vi "HFRR ADV v07.vi"() -> ()   [LabVIEW 2025] (continued)
                n1812 = local read "TEMPERATURE :"() -> (w2456:dbl)
                n1813 = local read "FRIC. FORCE :"() -> (w2457:dbl)
                n1814 = local read "HUMIDITY:"() -> (w2454:dbl)
                n1815 = Path To String(path="File Path") -> (string=w2524:string)
                n1816 = Number To Fractional String(number=w2463, width (-)=i16 10 ("precision (6)"), precision (6)=i16 5) -> (F-format string=w2482:string)  [unwired: 1 in]
                n1817 = Number To Fractional String(number=w2466, width (-)=i16 10 ("precision (6)"), precision (6)=i16 5) -> (F-format string=w2487:string)  [unwired: 1 in]
                n1818 = Number To Fractional String(number=w2469, width (-)=i16 10 ("precision (6)"), precision (6)=i16 5) -> (F-format string=w2490:string)  [unwired: 1 in]
                n1819 = Number To Fractional String(number=w2472, width (-)=i16 10 ("precision (6)"), precision (6)=i16 5) -> (F-format string=w2495:string)  [unwired: 1 in]
                n1820 = Number To Fractional String(number=w2475, width (-)=i16 10 ("precision (6)"), precision (6)=i16 5) -> (F-format string=w2498:string)  [unwired: 1 in]
                n1821 = Number To Fractional String(number=w2508, width (-)=i16 10 ("precision (6)"), precision (6)=i16 5) -> (F-format string=w2504:string)  [unwired: 1 in]
                n1822 = Number To Fractional String(number=w2452, width (-)=i16 10 ("precision (6)"), precision (6)=i16 5) -> (F-format string=w2515:string)  [unwired: 1 in]
                n1823 = local read "Com Port 2"() -> (w2458:refnum<visa-resource-name>)
                n1824 = local read "Com Port 1"() -> (w2459:refnum<visa-resource-name>)
                n1825 = Concatenate Strings(w2524, "\\" ("string")) -> (w2523:string)
                n1826 = Number To Fractional String(number=w2453, width (-)=i16 10 ("precision (6)"), precision (6)=i16 5) -> (F-format string=w2516:string)  [unwired: 1 in]
                n1827 = Number To Fractional String(number=w2455, width (-)=i16 10 ("precision (6)"), precision (6)=i16 5) -> (F-format string=w2543:string)  [unwired: 1 in]
                n1828 = Number To Fractional String(number=w2454, width (-)=i16 10 ("precision (6)"), precision (6)=i16 5) -> (F-format string=w2549:string)  [unwired: 1 in]
                n1829 = Number To Fractional String(number=w2456, width (-)=i16 10 ("precision (6)"), precision (6)=i16 5) -> (F-format string=w2555:string)  [unwired: 1 in]
                n1830 = Number To Fractional String(number=w2457, width (-)=i16 10 ("precision (6)"), precision (6)=i16 5) -> (F-format string=w2556:string)  [unwired: 1 in]
                n1831 = Concatenate Strings("[CHH]" ("string"), w2482, "-Humidity Dry" ("string"), "\r") -> (w2476:string)
                n1832 = Concatenate Strings("[CHG]" ("string"), w2487, "-Humidity Wet" ("string"), "\r") -> (w2477:string)
                n1833 = Concatenate Strings("[CHD]" ("string"), w2498, "-Power +" ("string"), "\r") -> (w2480:string)
                n1834 = Concatenate Strings("[CHC]" ("string"), w2504, "-Language Selection" ("string"), "\r") -> (w2501:string)
                n1835 = Concatenate Strings("[CHA]" ("string"), w2515, "- Stroke Gain" ("string"), "\r") -> (w2509:string)
                n1836 = Concatenate Strings("[CHF]" ("string"), w2490, "-Heater" ("string"), "\r") -> (w2478:string)
                n1837 = Concatenate Strings("[CHE]" ("string"), w2495, "-Power_" ("string"), "\r") -> (w2479:string)
                n1838 = Concatenate Strings("[CH8]" ("string"), w2516, "- Displacement Gain" ("string"), "\r") -> (w2519:string)
                n1839 = Concatenate Strings("[CH7]" ("string"), w2523, "- file path" ("string"), "\r") -> (w2526:string)
                n1840 = Concatenate Strings("[CH6]" ("string"), w2458, "- Visa Due" ("string"), "\r") -> (w2527:string)
                n1841 = Concatenate Strings("[CH5]" ("string"), w2459, "- Visa Uno" ("string"), "\r") -> (w2532:string)
                n1842 = Concatenate Strings("[CH4]" ("string"), w2543, " - AIR TEMP" ("string"), "\r") -> (w2539:string)
                n1843 = Concatenate Strings("[CH3]" ("string"), w2549, " - Humidity" ("string"), "\r") -> (w2546:string)
                n1844 = Concatenate Strings("[CH2]" ("string"), w2555, " - TEMPERATURE" ("string"), "\r") -> (w2553:string)
                n1845 = Concatenate Strings("[CH1]" ("string"), w2556, " - FF" ("string"), "\r") -> (w2554:string)
                n1846 = Concatenate Strings(w2554, w2553, w2546, w2539, w2532, w2527, w2526, w2519, w2509, w2501, w2480, w2479, w2478, w2477, w2476) -> (w2460:string)
                "gain" <- w2460
              }
              frame #1 {
                n1847 = local read "Camera Port :"() -> (w2568:string)
                n1848 = local read "C3 :"() -> (w2576:refnum<visa-resource-name>)
                n1849 = local read "TEMP INTERCEPT:"() -> (w2577:dbl)
                n1850 = local read "AIR TEMP INTERCEPT:"() -> (w2578:dbl)
                n1851 = Concatenate Strings("[CH8]" ("string"), w2568, "- Visa Camera" ("string"), "\r") -> (w2567:string)
                n1852 = Concatenate Strings("[CH7]" ("string"), w2576, "- Visa Humidity" ("string"), "\r") -> (w2572:string)
                n1853 = Number To Fractional String(number=w2577, width (-)=i16 10 ("precision (6)"), precision (6)=i16 5) -> (F-format string=w2595:string)  [unwired: 1 in]
                n1854 = local read "Com Port 3"() -> (w2579:refnum<visa-resource-name>)
                n1855 = Number To Fractional String(number=w2578, width (-)=i16 10 ("precision (6)"), precision (6)=i16 5) -> (F-format string=w2602:string)  [unwired: 1 in]
                n1856 = Concatenate Strings("[SNO]" ("string"), "S.NO", "-" ("string"), "\r") -> (w2587:string)
                n1857 = Concatenate Strings("[CHK]" ("string"), w2595, "-TEMP INTERCEPT" ("string"), "\r") -> (w2591:string)
                n1858 = Concatenate Strings("[CHJ]" ("string"), w2602, "-AIR TEMP INTERCEPT" ("string"), "\r") -> (w2592:string)
                n1859 = Concatenate Strings("[CHL]" ("string"), w2579, "- Visa humid" ("string"), "\r") -> (w2582:string)
                n1860 = String To Path(string="C:\\LAB-IQ\\calibrate WO 2465.dcf") -> (path=w2580:path)
                n1861 = Concatenate Strings(w2607, w2592, w2591, w2587, w2582, w2572, w2567) -> (w2606:string)
                n1862 = call <vilib>:"Write Characters To File.vi"("append to file? (new file:F)"=FALSE, "character string"=w2606, "file path (dialog if empty)"=w2580) -> ()  [unwired: 2 in, 1 out]
              }
              frame #2 {
                n1863 = local write "Lan flag"(0.0 ("Lan flag")) -> ()
                n1864 = local write "conststatus"(0.0 ("rpm value : 2")) -> ()
                n1865 = local write "SAVE"(FALSE ("OK Button 14")) -> ()
                n1866 = local write "SAVE 2"(FALSE ("SAVE 2")) -> ()
              }
            }
          }
        }
        n1867 = property on="Tab Control 7" class="TabCtl (strict)"("Disabled"=w2247) -> ()  [unwired: 2 in, 2 out]
        n1868 = property on="TEMP INTERCEPT:" class="DigNum (strict)"("Disabled"=w2247) -> ()  [unwired: 2 in, 2 out]
        n1869 = property on="AIR TEMP INTERCEPT:" class="DigNum (strict)"("Disabled"=w2247) -> ()  [unwired: 2 in, 2 out]
        n1870 = property on="DISPLACEMENT :" class="DigNum (strict)"("Disabled"=w2247) -> ()  [unwired: 2 in, 2 out]
        n1871 = property on="STROKE GAIN :" class="DigNum (strict)"("Disabled"=w2247) -> ()  [unwired: 2 in, 2 out]
        n1872 = property on="CH-HUMIDITY DRY" class="DigNum (strict)"("Disabled"=w2247) -> ()  [unwired: 2 in, 2 out]
        n1873 = property on="CH-HUMIDITY WET" class="DigNum (strict)"("Disabled"=w2247) -> ()  [unwired: 2 in, 2 out]
        n1874 = property on="CH-HEATER" class="DigNum (strict)"("Disabled"=w2247) -> ()  [unwired: 2 in, 2 out]
        n1875 = property on="CH-POWER -" class="DigNum (strict)"("Disabled"=w2247) -> ()  [unwired: 2 in, 2 out]
        n1876 = property on="CH-POWER +" class="DigNum (strict)"("Disabled"=w2247) -> ()  [unwired: 2 in, 2 out]
        n1877 = property on="Language Selection" class="Enum (strict)"("Visible"=w2246) -> ()  [unwired: 2 in, 2 out]
        n1878 = property on="AIR TEMPERATURE :" class="DigNum (strict)"("Disabled"=w2247) -> ()  [unwired: 2 in, 2 out]
        n1879 = property on="HUMIDITY:" class="DigNum (strict)"("Disabled"=w2247) -> ()  [unwired: 2 in, 2 out]
        n1880 = property on="FRIC. FORCE :" class="DigNum (strict)"("Disabled"=w2247) -> ()  [unwired: 2 in, 2 out]
        n1881 = property on="TEMPERATURE :" class="DigNum (strict)"("Disabled"=w2247) -> ()  [unwired: 2 in, 2 out]
        n1882 = property on="SPEED OUT:" class="DigNum (strict)"("Disabled"=w2247) -> ()  [unwired: 2 in, 2 out]
      }
    }
    n1883 = case shown="False" w1641 {
      frame False {
        n1884 = local read "stopT"() -> (w2619:bool)
        n1885 = case shown="True" w2619 {
          frame False {
          }
          frame True {
            n1886 = local write "stopT"(FALSE) -> ()
          }
        }
      }
      frame True {
        "stopT" <- TRUE
      }
    }
    n1887 = case shown="True" w1629 {
      frame False {
        n1888 = property on="Password 2" class="Str"("Visible"=FALSE) -> ()  [unwired: 2 in, 2 out]
        n1889 = local write "Password 2"("" ("Password")) -> ()
      }
      frame True {
        n1890 = property on="Password 2" class="Str"("Visible"=TRUE) -> ()  [unwired: 2 in, 2 out]
        n1891 = Equal?(x="Password 2", y="HFRR1234") -> (x = y?=w1761:bool)
        n1892 = case shown="True" w1761 {
          tunnel: "Password 2" -> [w1764 _]
          frame False {
            n1893 = String Length(string=w1764) -> (length=w1765:i32)
            n1894 = Greater Than 0?(x=w1765) -> (x > 0?=w1763:bool)
            n1895 = case shown="False" w1763 {
              frame False {
                n1896 = property on="Password 2" class="Str"("Caption.Text"="Password (Advance Setting)") -> ()  [unwired: 2 in, 2 out]
              }
              frame True {
                n1897 = property on="Password 2" class="Str"("Caption.Text"="Incorrect Password!") -> ()  [unwired: 2 in, 2 out]
              }
            }
          }
          frame True {
            (unwired) T26."Advance" ("Main Dashboard Buttons")
            n1898 = local write "EDIT 2"(FALSE ("EDIT 2")) -> ()
            n1899 = local write "Password 2"("" ("Password")) -> ()
            n1900 = local write "Main Tab"(T2."Advance" ("Main Tab")) -> ()
            n1901 = local write "Main Dashboard Buttons"(T1."Advance" ("Main Dashboard Buttons")) -> ()
          }
        }
      }
    }
    n1902 = disable-structure shown="Disabled" {
      disable-tunnel: [w1656 _] -> w1622
      disable-tunnel: [w1655 _] -> w1620
      frame Disabled {
        n1903 = local read "Temperature before test"() -> (w1649:dbl)
        n1904 = local read "Temperature after test"() -> (w1662:dbl)
        n1905 = Add(x=231.864, y=w1662) -> (x+y=w1659:dbl)
        n1906 = Add(x=231.864, y=w1649) -> (x+y=w1646:dbl)
        n1907 = case shown="True" "Save Results" {
          frame False {
          }
          frame True {
            w1678 = "\r"
            n1908 = local write "Save Results"(FALSE ("OK Button 5")) -> ()
            n1909 = local read "Temperature before test"() -> (w1716:dbl)
            n1910 = local read "Temperature after test"() -> (w1718:dbl)
            n1911 = local read "Humidity before test"() -> (w1715:dbl)
            n1912 = local read "Humidity after test"() -> (w1717:dbl)
            n1913 = local read "WS1.4"() -> (w1722:dbl)
            n1914 = local read "AVP"() -> (w1720:dbl)
            n1915 = Number To Fractional String(number=w1722, width (-)=i16 6, precision (6)=i16 1) -> (F-format string=w1682:string)  [unwired: 1 in]
            n1916 = local read "MWSD"() -> (w1719:dbl)
            n1917 = local read "String"() -> (w1711:string)
            n1918 = local read "FILE"() -> (w1714:string)
            n1919 = local read "HCF"() -> (w1721:dbl)
            n1920 = Number To Fractional String(number=w1718, width (-)=i16 6, precision (6)=i16 1) -> (F-format string=w1696:string)  [unwired: 1 in]
            n1921 = Number To Fractional String(number=w1717, width (-)=i16 6, precision (6)=i16 1) -> (F-format string=w1700:string)  [unwired: 1 in]
            n1922 = Number To Fractional String(number=w1720, width (-)=i16 6, precision (6)=i16 3) -> (F-format string=w1689:string)  [unwired: 1 in]
            n1923 = Number To Fractional String(number=w1716, width (-)=i16 6, precision (6)=i16 1) -> (F-format string=w1704:string)  [unwired: 1 in]
            n1924 = Number To Fractional String(number=w1715, width (-)=i16 6, precision (6)=i16 1) -> (F-format string=w1707:string)  [unwired: 1 in]
            n1925 = Concatenate Strings(w1711, w1714) -> (w1733:string)
            n1926 = Number To Fractional String(number=w1721, width (-)=i16 6, precision (6)=i16 2) -> (F-format string=w1687:string)  [unwired: 1 in]
            n1927 = Number To Fractional String(number=w1719, width (-)=i16 6, precision (6)=i16 1) -> (F-format string=w1693:string)  [unwired: 1 in]
            n1928 = Concatenate Strings("(" ("string"), w1682, ")Microns" ("string")) -> (w1681:string)
            n1929 = local read "REMARKS"() -> (w1713:string)
            "REMARKS 2" <- w1713
            n1930 = Concatenate Strings(w1687, ")" ("string")) -> (w1685:string)
            n1931 = Concatenate Strings("(" ("string"), w1707, " ) % RH," ("string")) -> (w1708:string)
            n1932 = Concatenate Strings("(" ("string"), w1689, ")  kPa," ("string")) -> (w1679:string)
            n1933 = Concatenate Strings("(" ("string"), w1693, ")  Microns," ("string")) -> (w1692:string)
            n1934 = Concatenate Strings("(" ("string"), w1696, ")  Deg C ," ("string")) -> (w1695:string)
            n1935 = Concatenate Strings("(" ("string"), w1700, " ) % RH," ("string")) -> (w1699:string)
            n1936 = Concatenate Strings("(" ("string"), w1704, ")  Deg C ," ("string")) -> (w1703:string)
            n1937 = Concatenate Strings(w1733, ".dwm" ("Substring")) -> (w1731:string)
            n1938 = String To Path(string=w1731) -> (path=w1730:path)
            n1939 = Concatenate Strings(w1713, w1678, " Humidity before test= " ("Substring"), w1708, w1678, " Temperature before test = " ("Substring"), w1703, w1678, " Humidity after test= " ("Substring"), w1699, w1678, "Temperature after test = " ("Substring"), w1695, w1678, "MSD = " ("Substring"), w1692, w1678, "  AVP = " ("Substring"), w1679, w1678, "  HCF                     =( " ("Substring"), w1685, w1678, " WS1.4                  = " ("Substring"), w1681, w1678) -> (w1677:string)
            "data" <- w1677
            n1940 = call <vilib>:"Write Characters To File.vi"("append to file? (new file:F)"=FALSE, "character string"=w1677, "file path (dialog if empty)"=w1730) -> ()  [unwired: 2 in, 1 out]
            n1941 = Match Pattern(string=w1677, regular expression="!") -> (after substring=→"export":string)  [unwired: 1 in, 3 out]
          }
        }
        n1942 = Divide(x=1705.984, y=w1659) -> (x/y=w1660:dbl)
        n1943 = Divide(x=1705.984, y=w1646) -> (x/y=w1647:dbl)
        n1944 = local read "Humidity before test"() -> (w1651:dbl)
        n1945 = local read "Humidity after test"() -> (w1664:dbl)
        n1946 = Subtract(x=8.017352 ("y"), y=w1660) -> (x-y=w1667:dbl)
        n1947 = Subtract(x=8.017352 ("y"), y=w1647) -> (x-y=w1673:dbl)
        n1948 = expression code="10**y"(w1667) -> (w1666:dbl)
        n1949 = expression code="10**y"(w1673) -> (w1653:dbl)
        n1950 = Multiply(x=w1664, y=w1666) -> (x*y=w1665:dbl)
        n1951 = Multiply(x=w1651, y=w1653) -> (x*y=w1652:dbl)
        n1952 = Divide(x=w1665, y=750.0) -> (x/y=w1669:dbl)
        n1953 = Divide(x=w1652, y=750.0) -> (x/y=w1668:dbl)
        n1954 = Add(x=w1668, y=w1669) -> (x+y=w1670:dbl)
        n1955 = Divide(x=w1670, y=2.0) -> (x/y=w1672:dbl)
        n1956 = local write "AVP"(w1672) -> ()
        n1957 = Subtract(x=1.4, y=w1672) -> (x-y=w1655:dbl)
        n1958 = local read "HCF"() -> (w1656:dbl)
      }
      frame Enabled {
      }
    }
    n1959 = case shown="\"Acquire\", Default" w1637 {
      frame "Acquire", Default {
        w2650 = 0.2 ("y")
        w2655 = 1.0 ("y")
        w2656 = 0.8 ("y")
        # "Elapsed time\ncof\nstroke\nAir temp\nTemp\nHumidity"
        n1960 = local read "RUN"() -> (w2659:bool)
        n1961 = local read "run replace"() -> (w2663:bool)
        n1962 = local read "run replace"() -> (w2662:bool)
        n1963 = stacked-sequence {
          frame #0 {
            n1964 = case shown="True" "RST FF" {
              frame False {
              }
              frame True {
                w2831 = 0.0 ("X Scale.Range:Maximum")
                n1965 = property on="Frictional Force ( N )" class="WFChart (strict)"("XScale.Maximum"=600.0 ("X Scale.Range:Maximum"), "XScale.Minimum"=w2831, "YScale.Maximum"=10.0 ("Y Scale.Range:Maximum"), "YScale.Minimum"=w2831) -> ()  [unwired: 2 in, 2 out]
              }
            }
          }
          frame #1 {
            n1966 = case shown="True" "RST TEMP" {
              frame False {
              }
              frame True {
                n1967 = property on="Temperature ( Deg C )" class="WFChart (strict)"("XScale.Minimum"=0.0 ("X Scale.Range:Minimum"), "XScale.Maximum"=600.0 ("X Scale.Range:Maximum"), "YScale.Minimum"=0.0 ("Y Scale.Range:Minimum"), "YScale.Maximum"=100.0 ("Y Scale.Range:Maximum")) -> ()  [unwired: 2 in, 2 out]
              }
            }
          }
          frame #2 {
            n1968 = case shown="True" "RSTCOF" {
              frame False {
              }
              frame True {
                n1969 = property on="Coefficient of Friction" class="WFChart (strict)"("XScale.Minimum"=0.0 ("X Scale.Range:Minimum"), "XScale.Maximum"=600.0 ("X Scale.Range:Maximum"), "YScale.Maximum"=1.0 ("X Scale.Range:Minimum"), "YScale.Minimum"=0.0 ("X Scale.Range:Minimum")) -> ()  [unwired: 2 in, 2 out]
              }
            }
          }
          frame #3 {
            n1970 = case shown="True" "RSTCOF 2" {
              frame False {
              }
              frame True {
                (unwired) 100.0 ("Y Scale.Range:Maximum")
                (unwired) 0.0 ("Y Scale.Range:Minimum")
                (unwired) 600.0 ("X Scale.Range:Maximum")
                (unwired) 0.0 ("X Scale.Range:Minimum")
              }
            }
          }
          frame #4 {
            n1971 = case shown="True" "RSTCOF 3" {
              frame False {
              }
              frame True {
                n1972 = property on="Electrical Contact Resistance ( % )" class="WFChart (strict)"("XScale.Minimum"=0.0 ("X Scale.Range:Minimum"), "XScale.Maximum"=600.0 ("X Scale.Range:Maximum"), "YScale.Minimum"=0.0 ("Y Scale.Range:Minimum"), "YScale.Maximum"=100.0 ("Y Scale.Range:Maximum")) -> ()  [unwired: 2 in, 2 out]
              }
            }
          }
        }
        n1973 = case shown="True" w2659 {
          frame False {
            n1974 = local write "run replace"(FALSE ("run replace")) -> ()
          }
          frame True {
            "run replace" <- TRUE ("run replace")
          }
        }
        n1975 = disable-structure shown="Disabled" {
          frame Disabled {
            n1976 = local read "RUN"() -> (w2670:bool)
            n1977 = local read "Flag"() -> (w2673:dbl)
            n1978 = Not(x=w2670) -> (.not. x?=w2669:bool)
            n1979 = Equal?(x=w2673, y=10.0) -> (x = y?=w2671:bool)
            n1980 = And(x=w2671, y=w2669) -> (x .and. y?=w2668:bool)
            n1981 = case shown="True" w2668 {
              frame False {
              }
              frame True {
                w2674 = FALSE ("Heater Button")
                n1982 = local write "Humidity"(w2674) -> ()
                n1983 = local write "Heater Button"(w2674) -> ()
              }
            }
          }
          frame Enabled {
          }
        }
        n1984 = local read "RUN"() -> (w2667:bool)
        n1985 = local read "Set Temp"() -> (w2629:dbl)
        n1986 = local read "SetTemp"() -> (w2631:dbl)
        n1987 = case shown="False" w2667 {
          tunnel: [FALSE ("TEST RUNNING") TRUE ("TEST RUNNING")] -> w2666
          frame False {
            w2850 = 0.0 ("Flag")
            n1988 = local write "Elapsed time"(0.0 ("elapsedtime")) -> ()
            n1989 = local write "Time Remaining"(w2850) -> ()
            n1990 = local write "Flag"(w2850) -> ()
            n1991 = local write "Remaining Time"(w2850) -> ()
          }
          frame True {
            n1992 = local write "Flag"(10.0 ("Flag")) -> ()
          }
        }
        n1993 = case shown="False" w2663 {
          frame False {
            n1994 = local read "zflag"() -> (→"zflag 2":dbl)
            n1995 = local write "FLAG 4"(0.0 ("FLAG")) -> ()
            n1996 = local write "yflag"(2.0 ("tflag")) -> ()
          }
          frame True {
            n1997 = local write "zflag"(3.0 ("zflag")) -> ()
            n1998 = local write "yflag"(1.0 ("tflag")) -> ()
          }
        }
        n1999 = local read "acq 2"() -> (w2661:bool)
        n2000 = local read "AIR TEMP"() -> (w2624:dbl)
        n2001 = local read "Amb temp"() -> (w2628:dbl)
        n2002 = case shown="True" "Save & Continue" {
          frame False {
          }
          frame True {
            "acq 2" <- TRUE ("acq 2")
          }
        }
        n2003 = local read "Set Rh"() -> (w2630:dbl)
        n2004 = Subtract(x=w2629, y=w2650) -> (x-y=w2652:dbl)
        n2005 = Add(x=w2629, y=w2650) -> (x+y=w2651:dbl)
        n2006 = Subtract(x=w2631, y=w2656) -> (x-y=w2658:dbl)
        n2007 = Add(x=w2631, y=w2656) -> (x+y=w2657:dbl)
        n2008 = And(x=w2661, y=w2662) -> (x .and. y?=w2660:bool)
        n2009 = disable-structure shown="Disabled" {
          frame Disabled {
            n2010 = case shown="True" {
              selector: _ -> [_ _]
              frame False {
              }
              frame True {
                n2011 = local read "zflag 2"() -> (w2732:dbl)
                n2012 = local read "yflag"() -> (w2734:dbl)
                n2013 = Equal?(x=w2732, y=3.0 ("tflag")) -> (x = y?=w2735:bool)
                n2014 = Equal?(x=w2734, y=2.0 ("tflag")) -> (x = y?=w2736:bool)
                n2015 = And(x=w2736, y=w2735) -> (x .and. y?=w2730:bool)
                n2016 = case shown="True" w2730 {
                  frame False {
                  }
                  frame True {
                    w2761 = 0.0 ("zflag")
                    n2017 = local write "zflag 2"(w2761) -> ()
                    n2018 = local write "zflag"(w2761) -> ()
                    n2019 = Delete(path (use dialog)=path "C:/LAB-IQ-NXT/WO 2449 TT.sig" ("file path (dialog if empty)")) -> (deleted path=w2760:path)  [unwired: 4 in, 2 out]
                    n2020 = Delete(path (use dialog)=path "C:/LAB-IQ-NXT/WO 2449 TRH.sig" ("file path (dialog if empty)")) -> (deleted path=w2755:path)  [unwired: 4 in, 2 out]
                    n2021 = local read "SENSOR TIME"() -> (w2745:dbl)
                    n2022 = local read "SEN.RUN HRS"() -> (w2747:dbl)
                    n2023 = call <vilib>:"compatOverwrite.vi"("overwrite (F)"=TRUE) -> ("overwrite?"=w2737:T27)
                    n2024 = call <vilib>:"compatOverwrite.vi"("overwrite (F)"=TRUE) -> ("overwrite?"=w2741:T27)
                    n2025 = local read "Total No. of Tests"() -> (w2748:dbl)
                    n2026 = Add(x=w2745, y=w2747) -> (x+y=w2746:dbl)
                    "SEN.RUN HRS" <- w2746
                    n2027 = Open/Create/Replace File(file path (use dialog)=w2760, operation (0:open)=w2737) -> (refnum out=w2738:refnum<file>, error out=w2739:errorcluster)  [unwired: 4 in, 1 out]
                    n2028 = Open/Create/Replace File(file path (use dialog)=w2755, operation (0:open)=w2741) -> (refnum out=w2742:refnum<file>, error out=w2743:errorcluster)  [unwired: 4 in, 1 out]
                    n2029 = Deny Access(4:w2739, 6:T24."deny none" ("deny mode (2)"), 7:w2738) -> (3:w2759:refnum<file>)  [unwired: 1 out]
                    n2030 = Deny Access(4:w2743, 6:T24."deny none" ("deny mode (2)"), 7:w2742) -> (3:w2751:refnum<file>)  [unwired: 1 out]
                    n2031 = Number To Decimal String(number=w2748) -> (decimal integer string=w2756:string)  [unwired: 1 in]
                    n2032 = Number To Decimal String(number=w2746) -> (decimal integer string=w2752:string)  [unwired: 1 in]
                    n2033 = Write to Binary File(file (use dialog)=w2759, data=w2756, 5:FALSE ("prepend array or string size? (T)")) -> ()  [unwired: 3 in, 3 out]
                    n2034 = Write to Binary File(file (use dialog)=w2751, data=w2752, 5:FALSE ("prepend array or string size? (T)")) -> ()  [unwired: 3 in, 3 out]
                  }
                }
              }
            }
          }
          frame Enabled {
          }
        }
        n2035 = Greater Or Equal?(x=w2624, y=15.0) -> (x >= y?=w2625:bool)
        "powstat" <- w2625
        n2036 = local read "Humidity ( %RH )"() -> (w2627:dbl)
        n2037 = Subtract(x=w2630, y=w2655) -> (x-y=w2653:dbl)
        n2038 = Add(x=w2630, y=w2655) -> (x+y=w2654:dbl)
        n2039 = In Range and Coerce(upper limit=w2657, x=w2628, lower limit=w2658) -> (In Range?=w2647:bool)  [unwired: 1 out]
        n2040 = local read "TEMP"() -> (w2626:dbl)
        n2041 = case shown="True" "Save & Continue" {
          frame False {
          }
          frame True {
            n2042 = local read "Operator ID"() -> (w3130:string)
            n2043 = local read "FILE"() -> (w3136:string)
            n2044 = String Length(string=w3130) -> (length=w3131:i32)
            n2045 = String Length(string=w3136) -> (length=w3134:i32)
            n2046 = Greater?(x=w3131, y=0) -> (0:w3129:bool)
            n2047 = Greater?(x=w3134, y=0) -> (0:w3133:bool)
            n2048 = And(x=w3133, y=w3129) -> (x .and. y?=w3128:bool)
            n2049 = case shown="True" w3128 {
              frame False {
                n2050 = stacked-sequence {
                  frame #0 {
                    n2051 = One Button Dialog(message="Please Enter a File Name and Operator ID to save data !", button name ("OK")="Ok") -> ()  [unwired: 1 out]
                  }
                  frame #1 {
                    n2052 = local write "Save & Continue"(FALSE ("OK Button")) -> ()
                  }
                }
                n2053 = local write "Save & Continue"(FALSE ("OK Button")) -> ()
              }
              frame True {
                n2054 = stacked-sequence {
                  frame #0 {
                    n2055 = local read "FILE"() -> (w3142:string)
                    n2056 = call "file check.vi"("file name in"=w3142) -> ("file name out"=w3141:string)  [unwired: 9 in, 1 out]
                    n2057 = call <vilib>:"Application Directory.vi"() -> ("Application Directory"=w3152:path)
                    n2058 = Build Path(base path=w3152, name or relative path="data") -> (appended path=w3151:path)
                    n2059 = call <vilib>:"Trim Whitespace.vi"("string"=w3141) -> ("trimmed string"=w3149:string)  [unwired: 1 in]
                    n2060 = call <vilib>:"Trim Whitespace.vi"("string"=w3141) -> ("trimmed string"=w3150:string)  [unwired: 1 in]
                    n2061 = List Folder(path=w3151) -> (folder names=w3147:string[])  [unwired: 3 in, 3 out]
                    n2062 = Match Pattern(string=w3149, regular expression="_(") -> (before substring=w3146:string)  [unwired: 1 in, 3 out]
                    n2063 = Equal?(x=w3147, y=w3146) -> (x = y?=w3155:bool[])
                    n2064 = for {
                      tunnel: w3147 -> [w3161] mode=indexing
                      tunnel: w3146 -> [w3159]
                      shift-right: [w3157] -> w3144
                      shift-left: bool[] [] -> [w3158]
                      n2065 = Match Pattern(string=w3161, regular expression="_(") -> (before substring=w3160:string)  [unwired: 1 in, 3 out]
                      n2066 = Equal?(x=w3160, y=w3159) -> (x = y?=w3156:bool)
                      n2067 = case shown="True" w3156 {
                        tunnel: w3156 -> [_ w3164]
                        tunnel: w3158 -> [w3163 w3166]
                        tunnel: [w3163 w3165] -> w3157
                        frame False {
                        }
                        frame True {
                          n2068 = Insert Into Array(array=w3166, new element=w3164) -> (w3165:bool[])  [unwired: 1 in]
                        }
                      }
                    }
                    n2069 = Or Array Elements(Boolean array=w3155) -> (logical OR=w3154:bool)
                    n2070 = Array Size(array=w3144) -> (size(s)=w3143:i32)
                    n2071 = case shown="True" w3154 {
                      tunnel: w3150 -> [_ w3174]
                      tunnel: w3143 -> [_ w3167]
                      frame False {
                      }
                      frame True {
                        n2072 = Number To Decimal String(number=w3167) -> (decimal integer string=w3170:string)  [unwired: 1 in]
                        n2073 = Search/Split String(string=w3174, search string/char (-)="_(" ("regular expression")) -> (substring before match=w3172:string)  [unwired: 1 in, 2 out]
                        n2074 = Concatenate Strings(w3172, "_(" ("regular expression"), w3170, ")" ("regular expression")) -> (w3168:string)
                        n2075 = local write "FILE"(w3168) -> ()
                      }
                    }
                  }
                  frame #1 {
                    w3176 = 0.0
                    w3189 = cluster{"y":dbl, dbl, "y":dbl}[] [] ("History Data")
                    w3190 = FALSE ("Heater Button")
                    (unwired) ")!" ("string")
                    (unwired) ")" ("string")
                    w3188 = dbl[] [] ("History Data")
                    w3194 = "\r"
                    # "C:\\WinDucom\\Data\\"
                    # "C:\\LAB-IQ-NXT\\data"
                    n2076 = local write "Humidity ( %RH )"(w3176) -> ()
                    n2077 = local write "Frequency ( Hz )"(w3176) -> ()
                    n2078 = local write "Stroke 3"(w3176) -> ()
                    n2079 = local write "Set Temp 2"(65.0 ("Set Temp 2")) -> ()
                    n2080 = local write "speedop"(0.0 ("PIDclk 2")) -> ()
                    n2081 = local write "AIR TEMP"(w3176) -> ()
                    n2082 = local write "Stroke 4"(w3176) -> ()
                    n2083 = local write "clk"(0.0 ("clk")) -> ()
                    n2084 = local write "COF 2"(w3176) -> ()
                    n2085 = local write "TEMP"(w3176) -> ()
                    n2086 = local write "ecr 3"(w3176) -> ()
                    n2087 = local write "FF 2"(w3176) -> ()
                    n2088 = local write "FF 3"(w3176) -> ()
                    n2089 = property on="Humidity ( %RH )" class="WFChart (strict)"("History Data"=w3188) -> ()  [unwired: 2 in, 2 out]
                    n2090 = property on="Temperature ( Deg C )" class="WFChart (strict)"("History Data"=w3188) -> ()  [unwired: 2 in, 2 out]
                    n2091 = property on="Electrical Contact Resistance ( % )" class="WFChart (strict)"("History Data"=w3188) -> ()  [unwired: 2 in, 2 out]
                    n2092 = property on="Frictional Force ( N )" class="WFChart (strict)"("History Data"=w3188) -> ()  [unwired: 2 in, 2 out]
                    n2093 = property on="Coefficient of Friction" class="WFChart (strict)"("History Data"=w3188) -> ()  [unwired: 2 in, 2 out]
                    n2094 = property on="Humidity ( %RH )" class="WFChart (strict)"("History Data"=w3188) -> ()  [unwired: 2 in, 2 out]
                    n2095 = property on="Temperature ( Deg C )" class="WFChart (strict)"("History Data"=w3188) -> ()  [unwired: 2 in, 2 out]
                    n2096 = property on="Electrical Contact Resistance ( % )" class="WFChart (strict)"("History Data"=w3188) -> ()  [unwired: 2 in, 2 out]
                    n2097 = property on="Frictional Force ( N )" class="WFChart (strict)"("History Data"=w3188) -> ()  [unwired: 2 in, 2 out]
                    n2098 = property on="Coefficient of Friction" class="WFChart (strict)"("History Data"=w3188) -> ()  [unwired: 2 in, 2 out]
                    n2099 = property on="Electrical Contact Resistance ( % )" class="WFChart (strict)"("History Data"=w3188) -> ()  [unwired: 2 in, 2 out]
                    n2100 = property on="Frictional Force ( N )" class="WFChart (strict)"("History Data"=w3188) -> ()  [unwired: 2 in, 2 out]
                    n2101 = property on="Coefficient of Friction" class="WFChart (strict)"("History Data"=w3188) -> ()  [unwired: 2 in, 2 out]
                    n2102 = property on="Stroke ( mm )" class="WFChart (strict)"("History Data"=w3189) -> ()  [unwired: 2 in, 2 out]
                    n2103 = property on="Stroke ( mm )" class="WFChart (strict)"("History Data"=w3189) -> ()  [unwired: 2 in, 2 out]
                    n2104 = local write "Humidity"(w3190) -> ()
                    n2105 = local write "Heater Button"(w3190) -> ()
                    n2106 = local read "FILE"() -> (w3184:string)
                    n2107 = disable-structure shown="Enabled" {
                      disable-tunnel: [w3229 _] -> w3175
                      frame Enabled {
                        n2108 = local read "NORMAL LOAD"() -> (w3229:dbl)
                      }
                      frame Disabled {
                      }
                    }
                    n2109 = call "file check.vi"("file name in"=w3184) -> ("error out"=w3187:errorcluster, "file name out"=w3181:string)  [unwired: 9 in]
                    n2110 = call "FILE PATH CREATION.vi"("error in"=w3187, "FILE NAME :"=w3181) -> ("FILE OUT"=w3180:path)  [unwired: 8 in, 1 out]
                    n2111 = Concatenate Strings(w3181, ".dgf" ("Substring")) -> (w3186:string)
                    n2112 = Concatenate Strings(w3181, ".duf" ("Substring")) -> (w3182:string)
                    n2113 = Multiply(x=w3175, y=1.0) -> (x*y=w3208:dbl)
                    n2114 = Build Path(base path=w3180, name or relative path=w3186) -> (appended path=w3179:path)
                    n2115 = Build Path(base path=w3180, name or relative path=w3182) -> (appended path=w3178:path)
                    n2116 = Number To Fractional String(number=w3208, width (-)=i16 5, precision (6)=i16 2) -> (F-format string=w3216:string)  [unwired: 1 in]
                    n2117 = local read "Fuel Discription :"() -> (w3204:string)
                    n2118 = local read "Batch Ref Num :"() -> (w3192:string)
                    n2119 = Get Date/Time String(date format (0)=enum16{"short", "long", "abbreviated"}."short") -> (date string=w3227:string, time string=w3224:string)  [unwired: 2 in]
                    n2120 = local read "Remarks :"() -> (w3203:string)
                    n2121 = Concatenate Strings("Load :- " ("Substring"), w3216, " grams ," ("Substring")) -> (w3215:string)
                    n2122 = local read "String 41"() -> (w3195:string)
                    n2123 = Concatenate Strings(w3192) -> (w3191:string)
                    n2124 = Concatenate Strings("tested by") -> (w3199:string)
                    n2125 = Concatenate Strings(w3204) -> (w3205:string)
                    n2126 = Concatenate Strings("(" ("Substring"), w3227, ")" ("Substring"), w3224) -> (w3197:string)
                    "concatenated string" <- w3197
                    n2127 = Concatenate Strings(w3203, "," ("string")) -> (w3202:string)
                    n2128 = Concatenate Strings("  TIME;      COF;       STROKE;     AIR TEMP;  TEMP;  HUMIDITY;  ECR; PID-OUT; FREQUENCY" ("Substring"), "\r") -> (w3211:string)
                    n2129 = Concatenate Strings(w3195, w3194, "Fuel Discription :-" ("Substring"), w3205, w3194, w3215, w3194, "Batch Ref Num :-" ("Substring"), w3191, w3194, " Remarks :- " ("Substring"), w3202, w3194, " Date :- " ("Substring"), w3197, w3194, "Tested By :-" ("Substring"), w3199) -> (w3209:string)
                    "REMARKS" <- w3209
                    n2130 = call <vilib>:"Write Characters To File.vi"("append to file? (new file:F)"=FALSE, "character string"=w3209, "file path (dialog if empty)"=w3178) -> ()  [unwired: 2 in, 1 out]
                    n2131 = call <vilib>:"Write Characters To File.vi"("append to file? (new file:F)"=FALSE, "character string"=w3211, "file path (dialog if empty)"=w3179) -> ()  [unwired: 2 in, 1 out]
                  }
                  frame #2 {
                    n2132 = local write "Cycles elapsed"(0 ("Cycles elapsed")) -> ()
                    n2133 = local write "cyclecount"(0 ("cyclecount")) -> ()
                    n2134 = local write "autostrtflg"(TRUE ("autostrtflg")) -> ()
                    n2135 = local write "Save"(FALSE ("Save")) -> ()
                    n2136 = local write "Save & Continue"(FALSE ("OK")) -> ()
                    n2137 = Get Date/Time In Seconds() -> (seconds since 1Jan1904=w3234:timestamp)
                    n2138 = To Double Precision Float(number=w3234) -> (double precision float=w3233:dbl)
                    n2139 = local write "acq timer"(w3233) -> ()
                    n2140 = One Button Dialog(message="Please ensure sample is mounted properly and machine is ready in all aspects for testing !", button name ("OK")="Ok") -> ()  [unwired: 1 out]
                  }
                  frame #3 {
                    n2141 = stacked-sequence {
                      frame #0 {
                        n2142 = local write "Main Dashboard Buttons"(T1."Dashboard" ("Main Dashboard Buttons")) -> ()
                        n2143 = local write "Main Tab"(T2."Acquire" ("Main Tab")) -> ()
                      }
                      frame #1 {
                        n2144 = local write "EVENT LOG"("" ("EVENT LOG")) -> ()
                      }
                      frame #2 {
                        n2145 = Wait (ms)(milliseconds to wait=u32 50) -> ()  [unwired: 1 out]
                      }
                      frame #3 {
                        n2146 = disable-structure shown="Disabled" {
                          frame Disabled {
                            n2147 = local read "EVENT LOG"() -> (w3246:string)
                            n2148 = call "Event Log.vi"("Content"="Test Details", "EVENT LOG"=w3246) -> ("EVENT LOG"=w3245:string)  [unwired: 8 in, 1 out]
                            n2149 = local write "EVENT LOG"(w3245) -> ()
                          }
                          frame Enabled {
                          }
                        }
                      }
                      frame #4 {
                        n2150 = Wait (ms)(milliseconds to wait=u32 50) -> ()  [unwired: 1 out]
                      }
                      frame #5 {
                        n2151 = local read "FILE"() -> (w3248:string)
                        n2152 = Concatenate Strings("File Name :" ("Content"), w3248) -> (w3249:string)
                        n2153 = local read "EVENT LOG"() -> (w3252:string)
                        n2154 = call "Event Log.vi"("Content"=w3249, "EVENT LOG"=w3252) -> ("EVENT LOG"=w3251:string)  [unwired: 8 in, 1 out]
                        n2155 = local write "EVENT LOG"(w3251) -> ()
                      }
                      frame #6 {
                        n2156 = Wait (ms)(milliseconds to wait=u32 50) -> ()  [unwired: 1 out]
                      }
                      frame #7 {
                        n2157 = local read "Batch Ref Num :"() -> (w3254:string)
                        n2158 = Concatenate Strings("Batch Ref No :" ("Content"), w3254) -> (w3255:string)
                        n2159 = local read "EVENT LOG"() -> (w3258:string)
                        n2160 = call "Event Log.vi"("Content"=w3255, "EVENT LOG"=w3258) -> ("EVENT LOG"=w3257:string)  [unwired: 8 in, 1 out]
                        n2161 = local write "EVENT LOG"(w3257) -> ()
                      }
                      frame #8 {
                        n2162 = Wait (ms)(milliseconds to wait=u32 50) -> ()  [unwired: 1 out]
                      }
                      frame #9 {
                        n2163 = local read "tested by"() -> (w3260:string)
                        n2164 = Concatenate Strings("Tested By :" ("Content"), w3260) -> (w3261:string)
                        n2165 = local read "EVENT LOG"() -> (w3264:string)
                        n2166 = call "Event Log.vi"("Content"=w3261, "EVENT LOG"=w3264) -> ("EVENT LOG"=w3263:string)  [unwired: 8 in, 1 out]
                        n2167 = local write "EVENT LOG"(w3263) -> ()
                      }
                      frame #10 {
                        n2168 = Wait (ms)(milliseconds to wait=u32 50) -> ()  [unwired: 1 out]
                      }
                      frame #11 {
                        n2169 = local read "TEST STANDARD"() -> (w3267:T3)
                        n2170 = case shown="\"ASTM D6079\", Default" w3267 {
                          tunnel: ["ASTM D6079" "ISO 12156" "CEC F-096-A-06" "Custom"] -> w3266
                          frame "ASTM D6079", Default {
                          }
                          frame "ISO 12156" {
                          }
                          frame "CEC F-096-A-06" {
                          }
                          frame "Custom" {
                          }
                        }
                        n2171 = Concatenate Strings("Test Standard :" ("Content"), w3266) -> (w3268:string)
                        n2172 = local read "EVENT LOG"() -> (w3271:string)
                        n2173 = call "Event Log.vi"("Content"=w3268, "EVENT LOG"=w3271) -> ("EVENT LOG"=w3270:string)  [unwired: 8 in, 1 out]
                        n2174 = local write "EVENT LOG"(w3270) -> ()
                      }
                      frame #12 {
                        n2175 = Wait (ms)(milliseconds to wait=u32 50) -> ()  [unwired: 1 out]
                      }
                      frame #13 {
                        n2176 = local read "Fuel Discription :"() -> (w3277:string)
                        n2177 = Concatenate Strings("Fuel Description :" ("Content"), w3277) -> (w3278:string)
                        n2178 = local read "EVENT LOG"() -> (w3281:string)
                        n2179 = call "Event Log.vi"("Content"=w3278, "EVENT LOG"=w3281) -> ("EVENT LOG"=w3280:string)  [unwired: 8 in, 1 out]
                        n2180 = local write "EVENT LOG"(w3280) -> ()
                      }
                      frame #14 {
                        n2181 = Wait (ms)(milliseconds to wait=u32 50) -> ()  [unwired: 1 out]
                      }
                      frame #15 {
                        n2182 = local read "Remarks :"() -> (w3283:string)
                        n2183 = Concatenate Strings("Remarks :" ("Content"), w3283) -> (w3284:string)
                        n2184 = local read "EVENT LOG"() -> (w3287:string)
                        n2185 = call "Event Log.vi"("Content"=w3284, "EVENT LOG"=w3287) -> ("EVENT LOG"=w3286:string)  [unwired: 8 in, 1 out]
                        n2186 = local write "EVENT LOG"(w3286) -> ()
                      }
                      frame #16 {
                        n2187 = Wait (ms)(milliseconds to wait=u32 50) -> ()  [unwired: 1 out]
                      }
                      frame #17 {
                        n2188 = local read "Operator ID"() -> (w3289:string)
                        n2189 = Concatenate Strings("Operator ID :" ("Content"), w3289) -> (w3291:string)
                        n2190 = local read "EVENT LOG"() -> (w3293:string)
                        n2191 = call "Event Log.vi"("Content"=w3291, "EVENT LOG"=w3293) -> ("EVENT LOG"=w3292:string)  [unwired: 8 in, 1 out]
                        n2192 = local write "EVENT LOG"(w3292) -> ()
                      }
                      frame #18 {
                        n2193 = Wait (ms)(milliseconds to wait=u32 50) -> ()  [unwired: 1 out]
                      }
                      frame #19 {
                        n2194 = disable-structure shown="Disabled" {
                          frame Disabled {
                            n2195 = local read "EVENT LOG"() -> (w3297:string)
                            n2196 = call "Event Log.vi"("Content"="Test Parameter", "EVENT LOG"=w3297) -> ("EVENT LOG"=w3296:string)  [unwired: 8 in, 1 out]
                            n2197 = local write "EVENT LOG"(w3296) -> ()
                          }
                          frame Enabled {
                          }
                        }
                      }
                      frame #20 {
                        n2198 = Wait (ms)(milliseconds to wait=u32 50) -> ()  [unwired: 1 out]
                      }
                      frame #21 {
                        n2199 = local read "Set Hz"() -> (w3301:dbl)
                        n2200 = Number To Fractional String(number=w3301, precision (6)=i16 2) -> (F-format string=w3300:string)  [unwired: 2 in]
                        n2201 = Concatenate Strings("Set Frequency [Hz] :" ("Content"), w3300) -> (w3303:string)
                        n2202 = local read "EVENT LOG"() -> (w3305:string)
                        n2203 = call "Event Log.vi"("Content"=w3303, "EVENT LOG"=w3305) -> ("EVENT LOG"=w3304:string)  [unwired: 8 in, 1 out]
                        n2204 = local write "EVENT LOG"(w3304) -> ()
                      }
                      frame #22 {
                        n2205 = Wait (ms)(milliseconds to wait=u32 50) -> ()  [unwired: 1 out]
                      }
                      frame #23 {
                        n2206 = local read "NORMAL LOAD"() -> (w3308:dbl)
                        n2207 = Number To Fractional String(number=w3308, precision (6)=i16 2) -> (F-format string=w3309:string)  [unwired: 2 in]
                        n2208 = Concatenate Strings("Applied Load [grams] :" ("Content"), w3309) -> (w3311:string)
                        n2209 = local read "EVENT LOG"() -> (w3313:string)
                        n2210 = call "Event Log.vi"("Content"=w3311, "EVENT LOG"=w3313) -> ("EVENT LOG"=w3312:string)  [unwired: 8 in, 1 out]
                        n2211 = local write "EVENT LOG"(w3312) -> ()
                      }
                      frame #24 {
                        n2212 = Wait (ms)(milliseconds to wait=u32 50) -> ()  [unwired: 1 out]
                      }
                      frame #25 {
                        n2213 = local read "Set Strk"() -> (w3316:dbl)
                        n2214 = Number To Fractional String(number=w3316, precision (6)=i16 2) -> (F-format string=w3317:string)  [unwired: 2 in]
                        n2215 = Concatenate Strings("Set Stroke [mm] :" ("Content"), w3317) -> (w3319:string)
                        n2216 = local read "EVENT LOG"() -> (w3321:string)
                        n2217 = call "Event Log.vi"("Content"=w3319, "EVENT LOG"=w3321) -> ("EVENT LOG"=w3320:string)  [unwired: 8 in, 1 out]
                        n2218 = local write "EVENT LOG"(w3320) -> ()
                      }
                      frame #26 {
                        n2219 = Wait (ms)(milliseconds to wait=u32 50) -> ()  [unwired: 1 out]
                      }
                      frame #27 {
                        n2220 = local read "Set Temp"() -> (w3324:dbl)
                        n2221 = Number To Fractional String(number=w3324, precision (6)=i16 2) -> (F-format string=w3325:string)  [unwired: 2 in]
                        n2222 = Concatenate Strings("Set Temperature [deg C] :" ("Content"), w3325) -> (w3327:string)
                        n2223 = local read "EVENT LOG"() -> (w3329:string)
                        n2224 = call "Event Log.vi"("Content"=w3327, "EVENT LOG"=w3329) -> ("EVENT LOG"=w3328:string)  [unwired: 8 in, 1 out]
                        n2225 = local write "EVENT LOG"(w3328) -> ()
                      }
                      frame #28 {
                        n2226 = Wait (ms)(milliseconds to wait=u32 50) -> ()  [unwired: 1 out]
                      }
                      frame #29 {
                        n2227 = local read "Set Rh"() -> (w3332:dbl)
                        n2228 = Number To Fractional String(number=w3332, precision (6)=i16 2) -> (F-format string=w3333:string)  [unwired: 2 in]
                        n2229 = Concatenate Strings("Set Humidity [%RH] :" ("Content"), w3333) -> (w3335:string)
                        n2230 = local read "EVENT LOG"() -> (w3337:string)
                        n2231 = call "Event Log.vi"("Content"=w3335, "EVENT LOG"=w3337) -> ("EVENT LOG"=w3336:string)  [unwired: 8 in, 1 out]
                        n2232 = local write "EVENT LOG"(w3336) -> ()
                      }
                      frame #30 {
                        n2233 = Wait (ms)(milliseconds to wait=u32 50) -> ()  [unwired: 1 out]
                      }
                      frame #31 {
                        n2234 = local read "test time"() -> (w3340:dbl)
                        n2235 = Number To Fractional String(number=w3340, precision (6)=i16 1) -> (F-format string=w3341:string)  [unwired: 2 in]
                        n2236 = Concatenate Strings("Test Duration [mins] :" ("Content"), w3341) -> (w3343:string)
                        n2237 = local read "EVENT LOG"() -> (w3345:string)
                        n2238 = call "Event Log.vi"("Content"=w3343, "EVENT LOG"=w3345) -> ("EVENT LOG"=w3344:string)  [unwired: 8 in, 1 out]
                        n2239 = local write "EVENT LOG"(w3344) -> ()
                      }
                      frame #32 {
                        w3346 = dbl[] [] ("History Data")
                        w3347 = cluster{"y":dbl, dbl, "y":dbl}[] [] ("History Data")
                        w3348 = FALSE ("Visible")
                        n2240 = property on="Stroke ( mm )" class="WFChart (strict)"("History Data"=w3347) -> ()  [unwired: 2 in, 2 out]
                        n2241 = property on="Humidity ( %RH )" class="WFChart (strict)"("History Data"=w3346) -> ()  [unwired: 2 in, 2 out]
                        n2242 = property on="Temperature ( Deg C )" class="WFChart (strict)"("History Data"=w3346) -> ()  [unwired: 2 in, 2 out]
                        n2243 = property on="Electrical Contact Resistance ( % )" class="WFChart (strict)"("History Data"=w3346) -> ()  [unwired: 2 in, 2 out]
                        n2244 = property on="Frictional Force ( N )" class="WFChart (strict)"("History Data"=w3346) -> ()  [unwired: 2 in, 2 out]
                        n2245 = property on="Coefficient of Friction" class="WFChart (strict)"("History Data"=w3346) -> ()  [unwired: 2 in, 2 out]
                        n2246 = property on="Coefficient of Friction" class="WFChart (strict)"("History Data"=w3346) -> ()  [unwired: 2 in, 2 out]
                        n2247 = property on="Electrical Contact Resistance ( % )" class="WFChart (strict)"("History Data"=w3346) -> ()  [unwired: 2 in, 2 out]
                        n2248 = property on="Frictional Force ( N )" class="WFChart (strict)"("History Data"=w3346) -> ()  [unwired: 2 in, 2 out]
                        n2249 = property on="Stroke ( mm )" class="WFChart (strict)"("History Data"=w3347) -> ()  [unwired: 2 in, 2 out]
                        n2250 = property on="Humidity ( %RH )" class="WFChart (strict)"("History Data"=w3346) -> ()  [unwired: 2 in, 2 out]
                        n2251 = property on="Temperature ( Deg C )" class="WFChart (strict)"("History Data"=w3346) -> ()  [unwired: 2 in, 2 out]
                        n2252 = property on="Service Password Log" class="Str"("Visible"=w3348) -> ()  [unwired: 2 in, 2 out]
                        n2253 = property on="Password 3" class="Clust (strict)"("Visible"=w3348) -> ()  [unwired: 2 in, 2 out]
                      }
                    }
                    "TEST FILE NAM,E SAVED" <- TRUE ("TEST FILE NAM,E SAVED")
                  }
                }
              }
            }
          }
        }
        n2254 = local write "Test \nStatus"(w2666) -> ()
        n2255 = local write "Save"(w2666) -> ()
        n2256 = local read "Main Tab"() -> (w2623:T2)
        n2257 = disable-structure shown="Disabled" {
          frame Disabled {
            n2258 = case shown="True" {
              selector: _ -> [_ _]
              frame False {
              }
              frame True {
                w2765 = TRUE ("Heater")
                n2259 = local write "Heater Button"(w2765) -> ()
                n2260 = local write "Humidity"(w2765) -> ()
                n2261 = local read "TEST STANDARD"() -> (w2763:T3)
                n2262 = local read "TEST STANDARD"() -> (w2768:T3)
                n2263 = Equal?(x=w2763, y=enum16{"ASTM D6079", "ISO 12156", "Custom"}."ASTM D6079" ("Test Standard")) -> (x = y?=w2762:bool)
                n2264 = Equal?(x=w2768, y=enum16{"ASTM D6079", "ISO 12156", "Custom"}."ISO 12156" ("Test Standard")) -> (x = y?=w2766:bool)
                n2265 = case shown="True" w2762 {
                  frame False {
                  }
                  frame True {
                    n2266 = local write "airtempflg"(TRUE ("airtempflg")) -> ()
                    n2267 = local write "Heater"(FALSE ("Heater")) -> ()
                  }
                }
                n2268 = case shown="True" w2766 {
                  frame False {
                  }
                  frame True {
                    n2269 = local write "airtempflg"(FALSE ("airtempflg")) -> ()
                    n2270 = local write "Heater"(TRUE ("Heater")) -> ()
                  }
                }
              }
            }
          }
          frame Enabled {
          }
        }
        n2271 = case shown="True" w2647 {
          tunnel: [FALSE ("RUN") TRUE ("RUN")] -> w2646
          tunnel: [_ 1] -> w2639
          frame False {
          }
          frame True {
          }
        }
        n2272 = In Range and Coerce(upper limit=w2651, x=w2626, lower limit=w2652) -> (In Range?=w2643:bool)  [unwired: 1 out]
        n2273 = In Range and Coerce(upper limit=w2654, x=w2627, lower limit=w2653) -> (In Range?=w2645:bool)  [unwired: 1 out]
        n2274 = case shown="True" w2643 {
          tunnel: [FALSE ("RUN") TRUE ("RUN")] -> w2642
          tunnel: [_ 3] -> w2637
          frame False {
          }
          frame True {
          }
        }
        n2275 = case shown="True" w2645 {
          tunnel: [FALSE ("RUN") TRUE ("RUN")] -> w2644
          tunnel: [_ 2] -> w2638
          frame False {
          }
          frame True {
          }
        }
        n2276 = case shown="\"Acquire\"" w2623 {
          tunnel: w2625 -> [_ w2856]
          frame Default {
            w2855 = 0.0 ("output")
            n2277 = local write "Frequency ( Hz )"(w2855) -> ()
            n2278 = local write "PID-out"(w2855) -> ()
          }
          frame "Acquire" {
            n2279 = stacked-sequence {
              frame #0 {
                n2280 = local read "Auto Start Test"() -> (w2861:bool)
                n2281 = case shown="True" w2861 {
                  tunnel: "RUN" -> [w2881 w2884]
                  tunnel: [w2881 w2883] -> w2862
                  frame False {
                  }
                  frame True {
                    n2282 = local read "Auto Start Temp"() -> (w2882:bool)
                    n2283 = Or(x=w2884, y=w2882) -> (x .or. y?=w2883:bool)
                  }
                }
                n2284 = local read "clk"() -> (w2880:dbl)
                n2285 = local read "Save"() -> (w2876:bool)
                n2286 = Equal?(x=w2880, y=0.0) -> (x = y?=w2877:bool)
                n2287 = And(x=w2877, y=w2876) -> (x .and. y?=w2878:bool)
                n2288 = Not(x="Engage") -> (.not. x?=w2867:bool)
                n2289 = case shown="True" w2862 {
                  tunnel: [0.0 w2901] -> w2859
                  frame False {
                    (unwired) TRUE ("Visible")
                    n2290 = local read "Auto Start Test"() -> (w2888:bool)
